vi "CreateQ.vi"(8 "error in (no error)":errorcluster, 9 "Initial QNames (Opt instead of Enum)":string[](array[string]), 10 "Type Def Enum (for datatype only)":variant) -> (0 "error out":errorcluster, 2 "dCVT QMH out":T1)   [LabVIEW 2020, in "QDict.lvlib"]
doc: "Developed by Kevin Thompson\nkevin@thompsonengineering.net\n\nCopyright 2021\nThompson Engineering, LLC"
uses:
  QDict.lvlib
  <vilib>/TELLC/Dynamic CVT API/TD Dynamic CVT DVR--ref.ctl
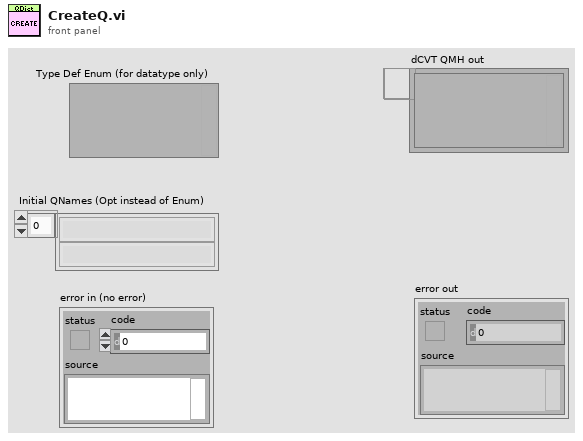
[diagram p1: front panel]
types:
  T1 = typedef "TD Dynamic CVT DVR--ref.ctl" = refnum<data-value>
  T2 = typedef "Type Descriptor Enumeration__ogtk.ctl" = enum8{"<Null>", "I8", "I16", "I32", "I64", "U8", "U16", "U32", "U64", "SGL", "DBL", "EXT", "CSG", "CDB", "CXT", "0x0F", "0x10", "0x11", "0x12", "0x13", "0x14", "Enum U8", "Enum U16", "Enum U32", "Enum U64", "SGL PQ", "DBL PQ", "EXT PQ", "CSG PQ", "CDB PQ", "CXT PQ", "0x1F", "0x20", "Boolean", "0x22", "0x23", "0x24", "0x25", "0x26", "0x27", "0x28", "0x29", "0x2A", "0x2B", "0x2C", "0x2D", "0x2E", "0x2F", "String", "0x31", "Path", "Pict", "0x34", "0x35", "0x36", "DAQ", "0x38", "0x39", "0x3A", "0x3B", "0x3C", "0x3D", "0x3E", "0x3F", "Array", "0x41", "0x42", "0x43", "0x44", "0x45", "0x46", "0x47", "0x48", "0x49", "0x4A", "0x4B", "0x4C", "0x4D", "0x4E", "0x4F", "Cluster", "0x51", "0x52", "Variant", "Waveform", "0x55", "0x56", "0x57", "0x58", "0x59", "0x5A", "0x5B", "0x5C", "0x5D", "0x5E", "0x5F", "0x60", "0x61", "0x62", "0x63", "0x64", "0x65", "0x66", "0x67", "0x68", "0x69", "0x6A", "0x6B", "0x6C", "0x6D", "0x6E", "0x6F", "Refnum"}
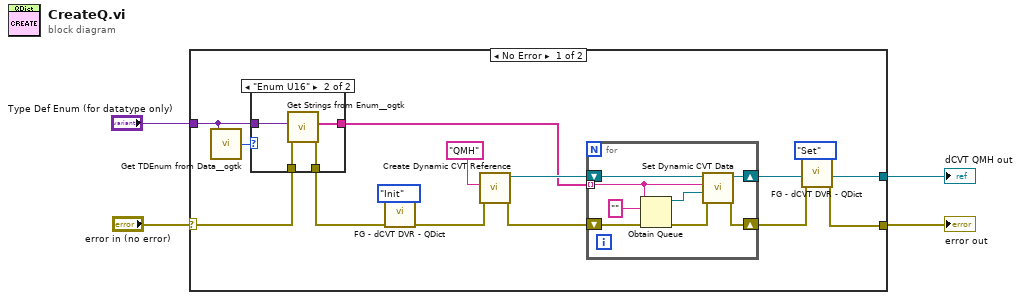
[diagram p0: block diagram]
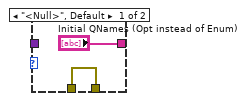
[diagram p2: hidden frame]
diagram:
  n1 = case shown="No Error" "error in (no error)" {
    selector: "error in (no error)" -> [w7 w34]
    tunnel: [w12 _] -> w4
    tunnel: [w10 w34] -> w3
    tunnel: "Type Def Enum (for datatype only)" -> [w8 _]
    frame No Error {
      n2 = call <userlib>:"Get TDEnum from Data__ogtk.vi"("Data"=w8) -> ("Type Descriptor Enumeration"=w9:T2)  [unwired: 4 in]
      n3 = case shown="\"Enum U16\"" w9 {
        tunnel: w8 -> [_ w25]
        tunnel: ["Initial QNames (Opt instead of Enum)" w24] -> w5
        tunnel: w7 -> [w20 w23]
        tunnel: [w20 w22] -> w6
        frame "<Null>", Default {
        }
        frame "Enum U16" {
          n4 = call <userlib>:"Get Strings from Enum__ogtk.vi"("error in (no error)"=w23, "Enum"=w25) -> ("error out"=w22:errorcluster, "Enum Strings"=w24:string[])  [unwired: 6 in, 2 out]
        }
      }
      n5 = call "FG - dCVT DVR - QDict.vi"("error in (no error)"=w6, "Action (Get)"=enum16{"Init", "Get", "Set"}."Init") -> ("error out"=w16:errorcluster)  [unwired: 7 in, 1 out]
      n6 = call <vilib>:"Create Dynamic CVT Reference.vi"("error in (no error)"=w16, "DictName"="QMH") -> ("error out"=w18:errorcluster, "dCVT DVR out"=w17:T1)  [unwired: 8 in]
      n7 = for {
        tunnel: w5 -> [w30] mode=indexing
        shift-right: [w28] -> w11
        shift-left: w18 -> [w32]
        shift-right: [w27] -> w14
        shift-left: w17 -> [w26]
        n8 = Obtain Queue(name (unnamed)=w30, element data type="", error in (no error)=w32) -> (queue out=w29:refnum<queue>, error out=w31:errorcluster)  [unwired: 2 in, 1 out]
        n9 = call <vilib>:"Set Dynamic CVT Data.vi"("error in (no error)"=w31, "value"=w29, "DataName"=w30, "dCVT DVR"=w26) -> ("error out"=w28:errorcluster, "dCVT DVR out"=w27:T1)  [unwired: 5 in, 1 out]
      }
      n10 = call "FG - dCVT DVR - QDict.vi"("dCVT QMH"=w14, "error in (no error)"=w11, "Action (Get)"=enum16{"Init", "Get", "Set"}."Set") -> ("dCVT QMH out"=w12:T1, "error out"=w10:errorcluster)  [unwired: 6 in]
    }
    frame Error {
    }
  }
  "dCVT QMH out" <- w4
  "error out" <- w3
